vi "LVMessageHandle.vi"() -> ()   [LabVIEW 2017]
panel:
  out "LVMsgHandle":u32
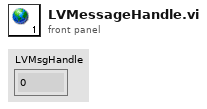
[diagram p1: front panel]
diagram:
